vi "CreateProxyObject.vi"(1 "object info":T1, 2 "remote object ref":refnum<class "G#Object.lvclass">, 3 "parameters":variant[](array[variant]), 5 "error in (no error)":errorcluster, 6 "connection ID":refnum<k5>, 8 "address":u32) -> (19 "error out":errorcluster)   [LabVIEW 2017, in "G#RemoteProxy.lvclass"]
doc: "Creates a proxy object."
uses:
  G#RemoteProxy.lvclass
  G#Object/utils/G#Object_ObjectInfoType.ctl
  G#Object/utils/G#Object_CreateMethod.ctl
  G#Object/G#Object.lvclass
  G#Object/utils/G#Object_ClassHierarchy.ctl
  G#DebugServer/G#DebugServer.lvclass
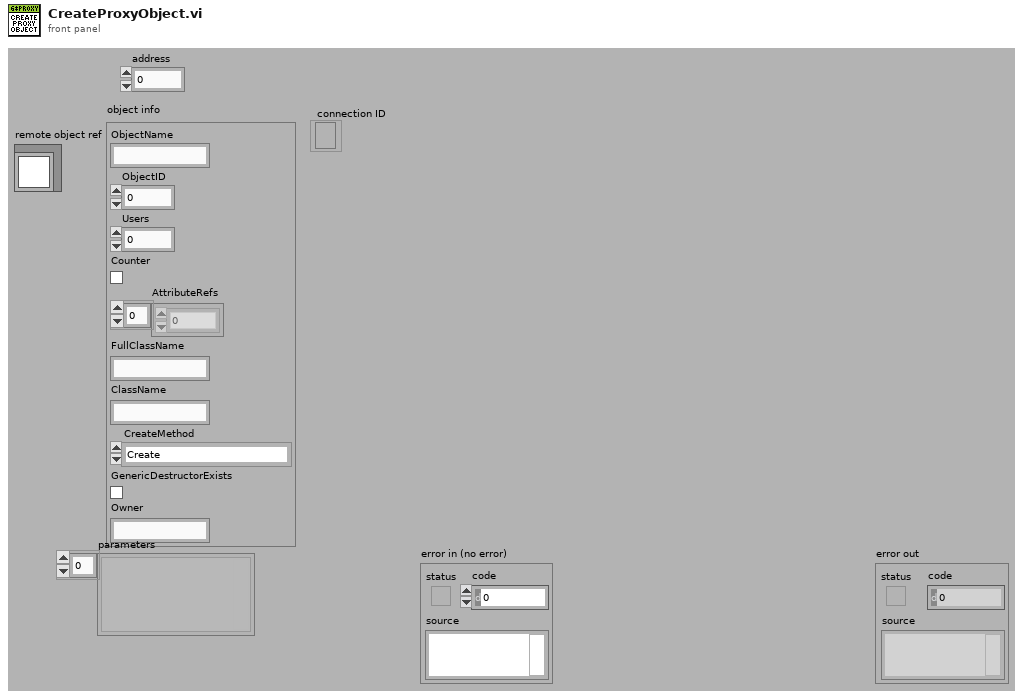
[diagram p1: front panel]
types:
  T1 = typedef "G#Object.lvclass/G#Object_ObjectInfoType.ctl" = cluster{"ObjectName":string, "ObjectID":u32, "Users":i32, "Counter":bool, "AttributeRefs":u32[], "FullClassName":string, "ClassName":string, "CreateMethod":T2, "GenericDestructorExists":bool, "Owner":string}
  T2 = typedef "G#Object.lvclass/G#Object_CreateMethod.ctl" = enum16{"Create", "Create or look up existing", "Look up existing"}
  T3 = typedef "G#Object.lvclass/G#Object_ClassHierarchy.ctl" = cluster{"ClassName":string, "FullClassName":string, "ClassPath":path, "IsLeaf":bool}
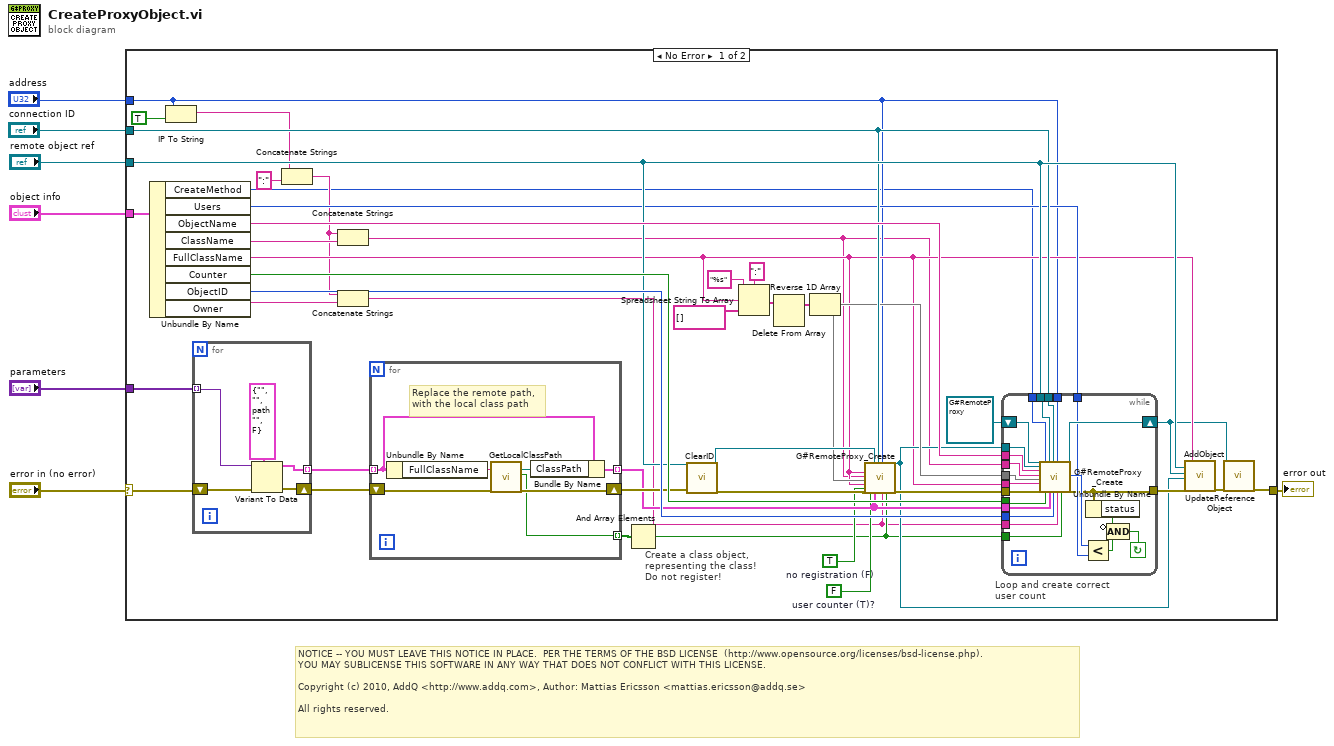
[diagram p0: block diagram]
diagram:
  # "NOTICE -- YOU MUST LEAVE THIS NOTICE IN PLACE.  PER THE TERMS OF THE BSD LICENSE  (http://www.opensource.org/licenses/bsd-license.php).\nYOU MAY SUBLICENSE THIS SOFTWARE IN ANY WAY THAT DOES NOT CONFLICT WITH THIS LICENSE.\n\nCopyright (c) 2010, AddQ <http://www.addq.com>, Author: Mattias Ericsson <mattias.ericsson@addq.se>\n\nAll rights reserved."
  n1 = case shown="No Error" "error in (no error)" {
    selector: "error in (no error)" -> [w42 w86]
    tunnel: [w10 w86] -> w6
    tunnel: "object info" -> [w37 _]
    tunnel: "remote object ref" -> [w31 _]
    tunnel: "parameters" -> [w43 _]
    tunnel: "address" -> [w22 _]
    tunnel: "connection ID" -> [w30 _]
    frame No Error {
      w27 = TRUE  # no registration (F)
      w28 = FALSE  # user counter (T)?
      # "Create a class object,\nrepresenting the class!\nDo not register!"
      # "Loop and create correct\nuser count"
      n2 = Unbundle By Name(w37) -> ("CreateMethod"=w8:T2, "Users"=w24:i32, "ObjectName"=w39:string, "ClassName"=w16:string, "FullClassName"=w23:string, "Counter"=w50:bool, "ObjectID"=w49:u32, "Owner"=w13:string)
      n3 = IP To String(1:TRUE ("dot notation? (F)"), 2:w22) -> (0:w20:string)
      n4 = for {
        tunnel: w43 -> [w75] mode=indexing
        shift-right: [w77] -> w40
        shift-left: w42 -> [w76]
        tunnel: [w74] -> w41 mode=indexing
        n5 = Variant To Data(error in=w76, type=T3 {"ClassName"="", "FullClassName"="", "ClassPath"=path "", "IsLeaf"=FALSE} ("ClassHierarchy"), Variant=w75) -> (data=w74:T3, error out=w77:errorcluster)
      }
      n6 = Concatenate Strings(w20, ":" ("string")) -> (w14:string)
      n7 = Concatenate Strings(w14, w16) -> (w15:string)
      n8 = Concatenate Strings(w14, w13) -> (w12:string)
      n9 = for {
        shift-right: [w80] -> w34
        shift-left: w40 -> [w83]
        tunnel: w41 -> [w85] mode=indexing
        tunnel: [w84] -> w29 mode=indexing
        tunnel: [w79] -> w18 mode=indexing
        # "Replace the remote path,\nwith the local class path"
        n10 = Unbundle By Name(w85) -> ("FullClassName"=w82:string)
        n11 = call "GetLocalClassPath.vi"("full class name"=w82, "error in (no error)"=w83) -> ("local class path"=w81:path, "found?"=w79:bool, "error out"=w80:errorcluster)  [unwired: 15 in]
        n12 = Bundle By Name(cluster=w85, "ClassPath"=w81) -> (w84:T3)
      }
      n13 = And Array Elements(Boolean array=w18) -> (logical AND=w17:bool)
      n14 = call "ClearID.vi"("G#DebugServer ref"=w31, "error in (no error)"=w34) -> ("G#DebugServer ref out"=w32:refnum<class "G#Object.lvclass">, "error out"=w33:errorcluster)  [unwired: 16 in]
      n15 = Spreadsheet String To Array(delimiter (Tab)=":", format string="%s", spreadsheet string=w23, array type (2D Dbl)=string[] []) -> (array=w45:string[])
      n16 = Delete From Array(array=w45) -> (array with subset deleted=w44:string[])  [unwired: 2 in, 1 out]
      n17 = Reverse 1D Array(array=w44) -> (reversed array=w26:string[])
      n18 = call "G#RemoteProxy_Create.vi"("object name"=w23, "class name"=w15, "lvlib hierarchy"=w26, "full class name"=w23, "no registration (F)"=w27, "error in (no error)"=w33, "user counter (T)?"=w28, "remote object ref"=w32, "class hierarchy"=w29, "connection ID"=w30, "address"=w22, "owner"=w12, "in memory?"=w17) -> ("reference out"=w25:refnum<class "G#RemoteProxy.lvclass">, "error out"=w35:errorcluster)  [unwired: 12 in, 1 out]
      n19 = while {
        tunnel: w15 -> [w60]
        tunnel: w50 -> [w63]
        tunnel: w49 -> [w65]
        tunnel: w12 -> [w66]
        tunnel: w23 -> [w62]
        tunnel: w26 -> [w61]
        tunnel: w35 -> [w71]
        tunnel: w29 -> [w64]
        tunnel: [w55] -> w36
        tunnel: w31 -> [w68]
        tunnel: w39 -> [w59]
        shift-right: [w72] -> w9
        shift-left: refnum<class "G#RemoteProxy.lvclass"> refnum ("reference out") -> [w73]
        tunnel: w22 -> [w70]
        tunnel: w30 -> [w69]
        tunnel: w25 -> [w67]
        tunnel: w24 -> [w57]
        tunnel: w17 -> [w56]
        tunnel: w8 -> [w51]
        stop <- w52 continue-if-true
        n20 = call "G#RemoteProxy_Create.vi"("reference in"=w73, "proxy class ref"=w67, "object name"=w59, "class name"=w60, "lvlib hierarchy"=w61, "full class name"=w62, "error in (no error)"=w71, "create method"=w51, "user counter (T)?"=w63, "remote object ref"=w68, "class hierarchy"=w64, "connection ID"=w69, "id"=w65, "address"=w70, "owner"=w66, "in memory?"=w56) -> ("reference out"=w72:refnum<class "G#RemoteProxy.lvclass">, "# of users"=w58:i32, "error out"=w55:errorcluster)  [unwired: 9 in]
        n21 = Less?(x=w58, y=w57) -> (x < y?=w53:bool)
        n22 = Unbundle By Name(w55) -> ("status"=w54:bool)
        n23 = Compound Arithmetic op=AND(invert w54, w53) -> (w52:bool)
      }
      n24 = call "AddObject.vi"("remote object ref"=w31, "proxy object ref"=w9, "proxy class object ref"=w25, "error in (no error)"=w36, "full class name"=w23) -> ("error out"=w11:errorcluster)  [unwired: 14 in]
      n25 = call "UpdateReferenceObject.vi"("reference in"=w9, "error in (no error)"=w11) -> ("error out"=w10:errorcluster)  [unwired: 16 in, 1 out]
    }
    frame Error {
    }
  }
  "error out" <- w6
